vi "Data_PSD_257.vi"() -> ()   [LabVIEW 2020]
uses:
  <vilib>/Utility/error.llb/DialogType.ctl
  <vilib>/Analysis/4window.llb/windowTd.ctl
  <vilib>/Analysis/NI_AALPro.lvlib
  <vilib>/measure/maspectr.llb/Power Spectrum and PSD Export Mode.ctl
  <vilib>/measure/NI_MAPro.lvlib
  <vilib>/sound2/lvsound2.llb/Sound File Info (path).vi
  <vilib>/sound2/lvsound2.llb/Sound File Read (DBL).vi
  <vilib>/sound2/lvsound2.llb/Sound File Read Open.vi
  <vilib>/Analysis/0measdsp.llb/Scaled Time Domain Window (DBL).vi
  <vilib>/measure/maspectr.llb/FFT Power Spectrum and PSD for 1 Chan.vi
panel:
  in  "Stop":bool
  out "Data Cursor":T1
  in  "File Path":path
  out "Max Amplitude":dbl
  out "Frequency Peak":dbl
  out "Signal":waveform(dbl)(graph)
  out "PSD of Signal":cluster{"f0":dbl, "df":dbl, "magnitude":dbl[]}(graph)
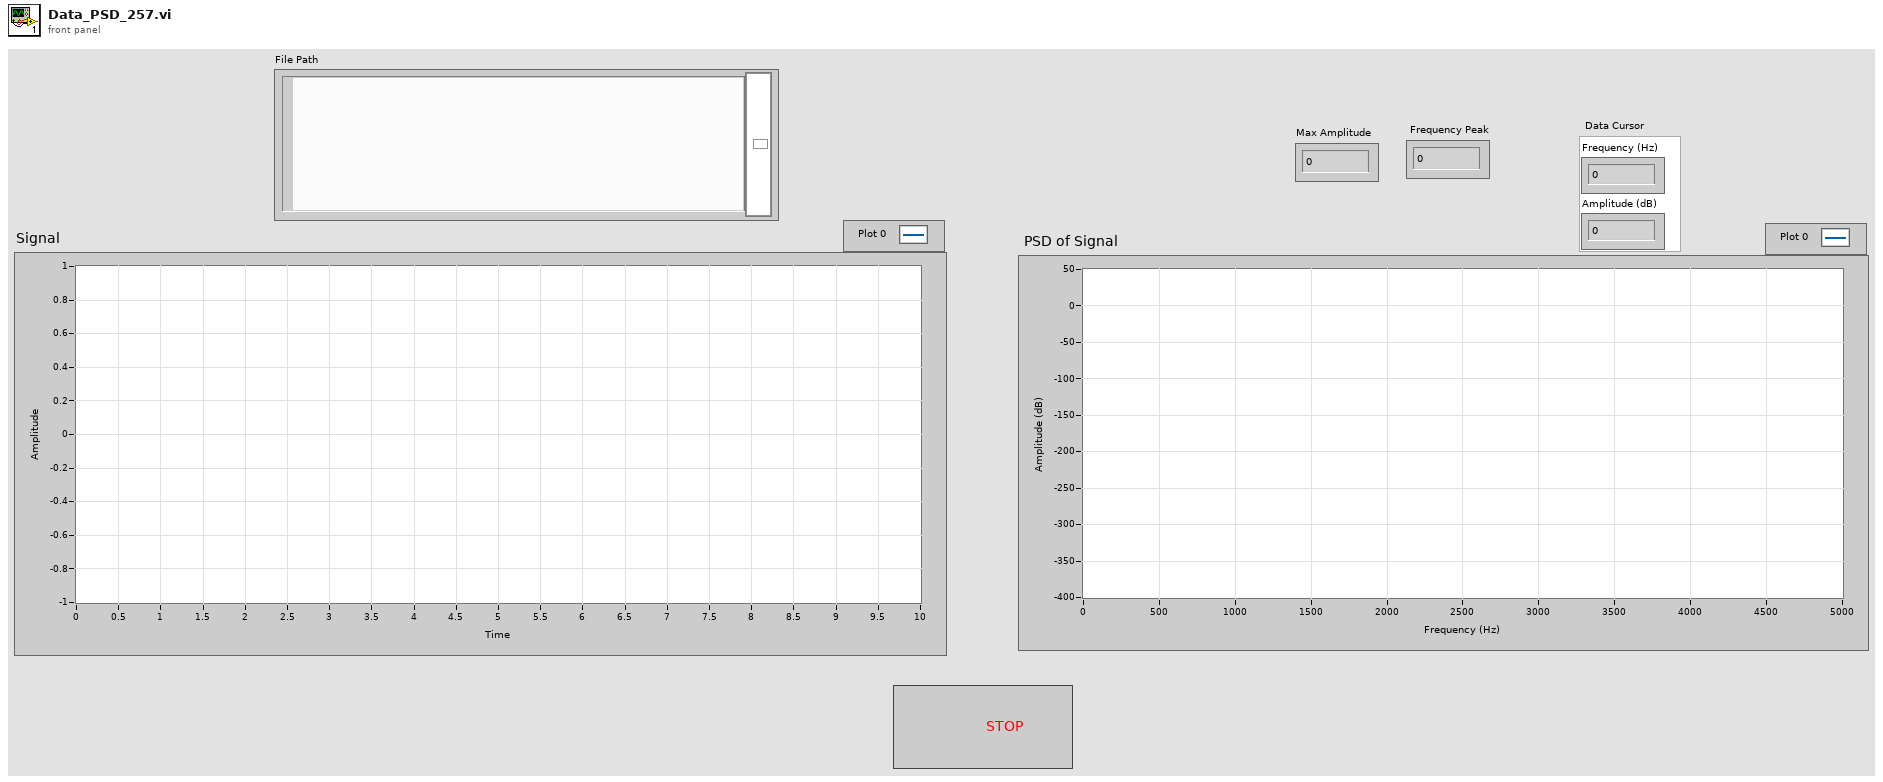
[diagram p1: front panel]
types:
  T1 = cluster{"Frequency (Hz)":dbl, "Amplitude (dB)":dbl}
  T2 = cluster{"Data":dbl[], "ctl":enum16{"Init", "Exit"}}
  T3 = typedef "DialogType.ctl" = u16
  T4 = typedef "NI_AALPro.lvlib/windowTd.ctl" = u32
  T5 = typedef "NI_MAPro.lvlib/Power Spectrum and PSD Export Mode.ctl" = u16
  T6 = typedef "LVPointDoubleTypeDef.ctl" = cluster{"Cursor X":dbl, "Cursor Y":dbl}
  T7 = typedef "Sound File Refnum.ctl" = refnum<file>
  T8 = typedef "LVRangeTypeDef.ctl" = cluster{"Minimum":dbl, "Maximum":dbl, "Increment":dbl, "Minor Increment":dbl, "Start":dbl}
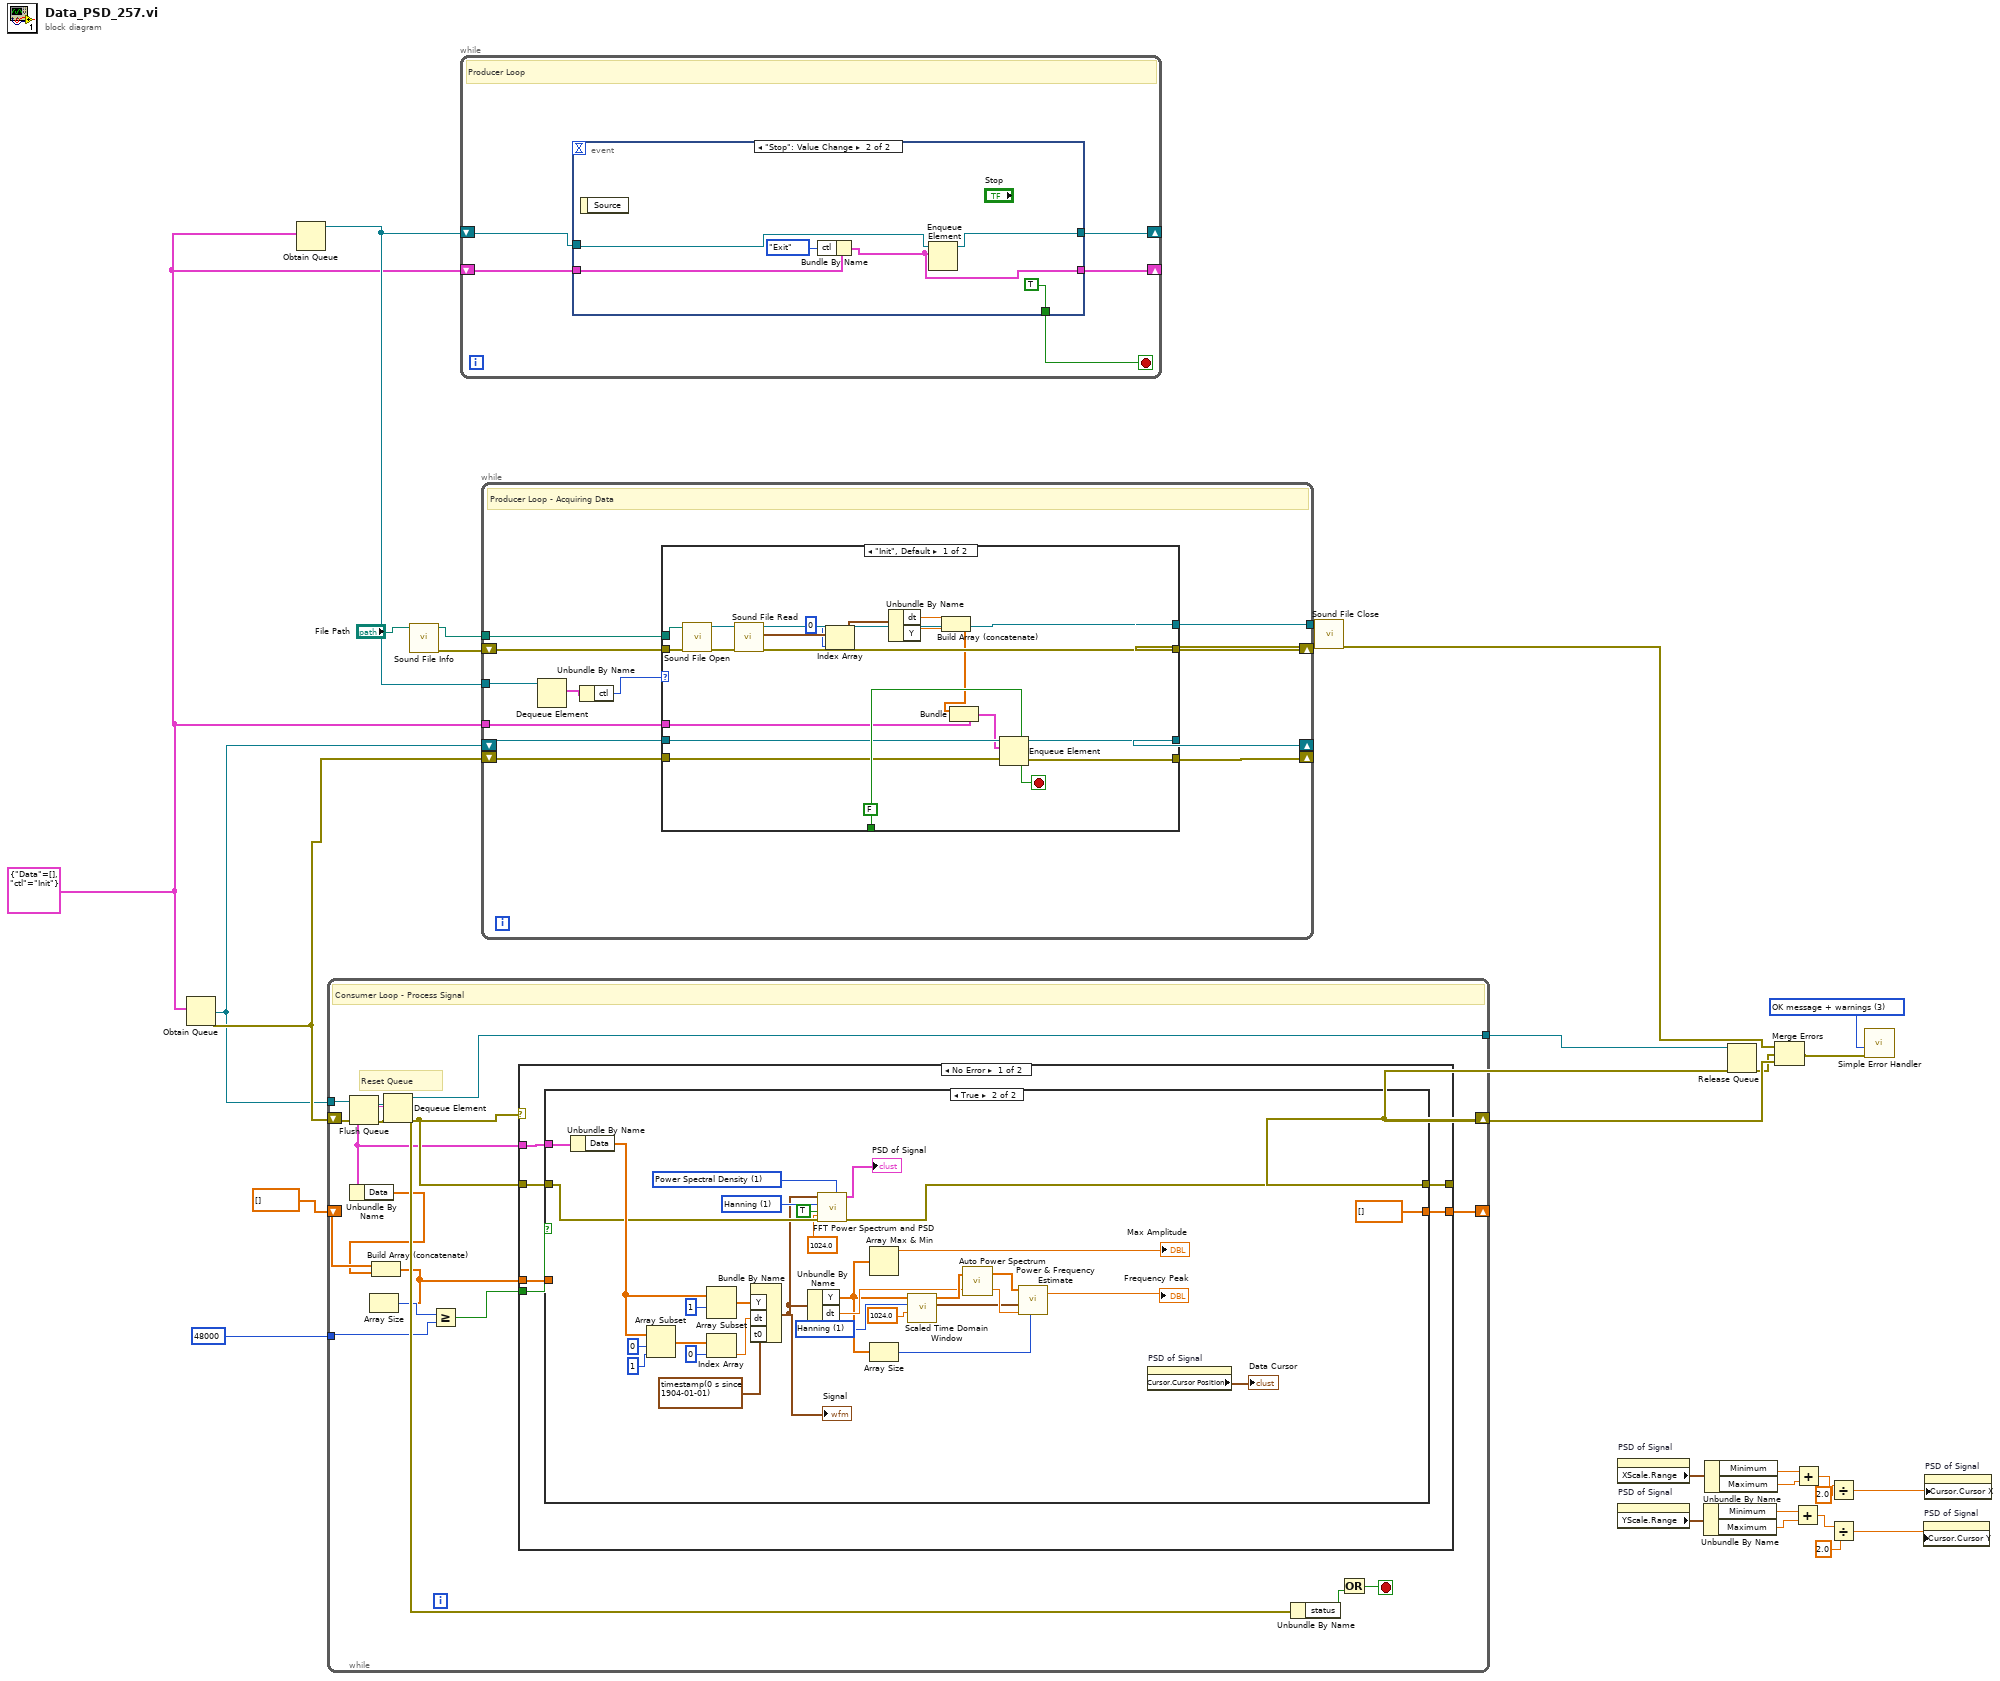
[diagram p0: block diagram]
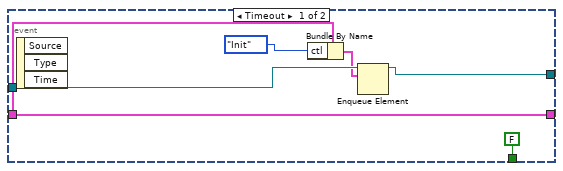
[diagram p2: hidden frame]
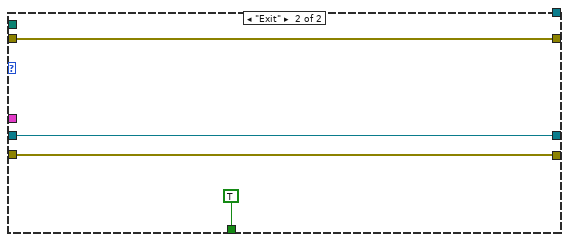
[diagram p3: hidden frame]
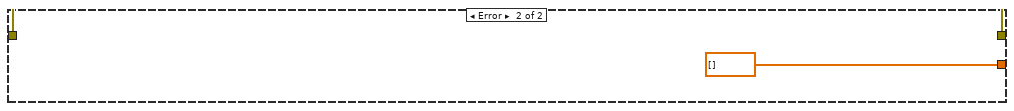
[diagram p5: hidden frame]
diagram:
  w1 = T2 {"Data"=[], "ctl"=enum."Init"}
  w29 = T3 3 items=["no dialog", "OK message", "continue or stop message", "OK message + warnings", "continue/stop + warnings"] ("type of dialog (OK msg:1)")
  n1 = Obtain Queue(element data type=w1) -> (queue out=w18:refnum<queue>, error out=w19:errorcluster)  [unwired: 3 in, 2 out]
  n2 = Obtain Queue(element data type=w1) -> (queue out=w2:refnum<queue>)  [unwired: 4 in, 2 out]
  n3 = while {
    tunnel: w18 -> [w43]
    shift-right: [w46] -> w26
    shift-left: w19 -> [w41]
    tunnel: [w39] -> w27
    tunnel: 48000 -> [w35]
    shift-right: [w31] -> _
    shift-left: dbl[] [] -> [w36]
    stop <- w44 stop-if-true
    # "Reset Queue"
    # "Consumer Loop - Process Signal"
    n4 = Flush Queue(queue=w43, error in (no error)=w41) -> (queue out=w42:refnum<queue>, error out=w40:errorcluster)  [unwired: 1 out]
    n5 = Dequeue Element(queue=w42, error in (no error)=w40) -> (queue out=w39:refnum<queue>, element=w37:T2, error out=w38:errorcluster)  [unwired: 2 out]
    n6 = Unbundle By Name(w37) -> ("Data"=w32:dbl[])
    n7 = Build Array (concatenate)(w36, w32) -> (w30:dbl[])
    n8 = Array Size(array=w30) -> (size(s)=w34:i32)
    n9 = Greater Or Equal?(x=w34, y=w35) -> (x >= y?=w33:bool)
    n10 = case shown="No Error" w38 {
      tunnel: w37 -> [w52 _]
      tunnel: [w47 w87] -> w46
      tunnel: w38 -> [w48 w87]
      tunnel: w33 -> [w51 _]
      tunnel: [w50 dbl[] []] -> w31
      tunnel: w30 -> [w49 _]
      frame No Error {
        n11 = case shown="True" w51 {
          tunnel: w52 -> [_ w67]
          tunnel: [w54 dbl[] []] -> w50
          tunnel: w49 -> [w54 _]
          tunnel: w48 -> [w53 w63]
          tunnel: [w53 w62] -> w47
          frame False {
          }
          frame True {
            w68 = T4 1 items=["Rectangle"=0, "Hanning"=1, "Hamming"=2, "Blackman-Harris"=3, "Exact Blackman"=4, "Blackman"=5, "Flat Top"=6, "4 Term B-Harris "=7, "7 Term B-Harris"=8, "Low Sidelobe"=9, "Blackman Nuttall"=11, "Triangle"=30, "Bartlett-Hanning"=31, "Bohman"=32, "Parzen"=33, "Welch"=34, "Kaiser"=60, "Dolph-Chebyshev"=61, "Gaussian"=62] ("window")
            w69 = T4 1 items=["Rectangle"=0, "Hanning"=1, "Hamming"=2, "Blackman-Harris"=3, "Exact Blackman"=4, "Blackman"=5, "Flat Top"=6, "4 Term B-Harris "=7, "7 Term B-Harris"=8, "Low Sidelobe"=9, "Blackman Nuttall"=11, "Triangle"=30, "Bartlett-Hanning"=31, "Bohman"=32, "Parzen"=33, "Welch"=34, "Kaiser"=60, "Dolph-Chebyshev"=61, "Gaussian"=62] ("window")
            w82 = T5 1 items=["Power Spectrum", "Power Spectral Density"] ("export mode")
            n12 = Unbundle By Name(w67) -> ("Data"=w66:dbl[])
            n13 = Array Subset(array=w66, index=0, length=1) -> (w78:dbl[])
            n14 = Array Subset(array=w66, index=1) -> (w79:dbl[])  [unwired: 1 in]
            n15 = Index Array(array=w78, index=0) -> (element=w76:dbl)
            n16 = Bundle By Name("Y"=w79, "dt"=w76, "t0"=timestamp(0 s since 1904-01-01)) -> (w55:waveform(dbl))  [unwired: 1 in]
            "Signal" <- w55
            n17 = Unbundle By Name(w55) -> ("Y"=w72:dbl[], "dt"=w81:dbl)
            n18 = call-poly <vilib>:"FFT Power Spectrum and PSD.vi"("window parameter"=1024.0, "export mode"=w82, "error in (no error)"=w63, "dB On (F)"=TRUE, "window"=w68, "time signal"=w55) -> ("error out"=w62:errorcluster, "Power Spectrum / PSD"=→"PSD of Signal":cluster{"f0":dbl, "df":dbl, "magnitude":dbl[]})  [unwired: 2 in, 2 out]
            n19 = Array Max & Min(array=w72) -> (max value=→"Max Amplitude":dbl)  [unwired: 3 out]
            n20 = Array Size(array=w72) -> (size(s)=w71:i32)
            n21 = call-poly <vilib>:"Scaled Time Domain Window.vi"("window parameter"=1024.0, "window"=w69, "X"=w72) -> ("window properties"=w70:cluster{"eq noise BW":dbl, "coherent gain":dbl}, "Windowed X"=w84:dbl[])  [unwired: 7 out]
            n22 = call <vilib>:"Auto Power Spectrum.vi"("dt"=w81, "Signal (V)"=w84) -> ("df"=w85:dbl, "Power Spectrum (V^2 rms)"=w73:dbl[])
            n23 = call <vilib>:"Power & Frequency Estimate.vi"("span"=w71, "df"=w85, "window constants"=w70, "Power Spectrum (V^2 rms)"=w73) -> ("est frequency peak"=→"Frequency Peak":dbl)  [unwired: 1 in, 2 out]
            n24 = property on="PSD of Signal" class="WFGraph (strict)"() -> ("Cursor.Cursor Position"=→"Data Cursor":T6)  [unwired: 2 in, 2 out]
          }
        }
      }
      frame Error {
      }
    }
    n25 = Unbundle By Name(w38) -> ("status"=w45:bool)
    n26 = Or(y=w45) -> (x .or. y?=w44:bool)  [unwired: 1 in]
  }
  n27 = call-poly <vilib>:"Sound File Info.vi"("path"="File Path") -> ("error out"=w22:errorcluster, "path out"=w23:path)  [unwired: 7 in, 2 out]
  n28 = while {
    shift-right: [w88] -> _
    shift-left: w1 -> [w91]
    shift-right: [w90] -> _
    shift-left: w2 -> [w92]
    stop <- w89 stop-if-true
    # "Producer Loop"
    n29 = event shown="[1] \"Stop\": Value Change" {
      selector: _ -> [_ _]
      dyn-events: _ -> [_ _]
      timeout: _ -> [_ _]
      tunnel: w92 -> [w98 w102]
      tunnel: w91 -> [w93 w104]
      tunnel: [w95 w101] -> w90
      tunnel: [FALSE TRUE] -> w89
      tunnel: [w93 w99] -> w88
      event Timeout {
        n30 = event-data() -> ()  [unwired: 1 in, 3 out]
        n31 = Bundle By Name(cluster=w93, "ctl"=enum16{"Init", "Exit"}."Init") -> (w96:T2)
        n32 = Enqueue Element(queue=w98, element=w96) -> (queue out=w95:refnum<queue>)  [unwired: 2 in, 2 out]
      }
      event "Stop": Value Change {
        n33 = event-data() -> ()  [unwired: 1 in, 1 out]
        n34 = Bundle By Name(cluster=w104, "ctl"=enum16{"Init", "Exit"}."Exit") -> (w99:T2)
        n35 = Enqueue Element(queue=w102, element=w99) -> (queue out=w101:refnum<queue>)  [unwired: 2 in, 2 out]
      }
    }
  }
  n36 = while {
    shift-right: [w116] -> _
    shift-left: w19 -> [w117]
    shift-right: [w111] -> w20
    shift-left: w22 -> [w113]
    tunnel: w23 -> [w114]
    tunnel: [w112] -> w21
    shift-right: [w109] -> _
    shift-left: w18 -> [w110]
    tunnel: w1 -> [w108]
    tunnel: w2 -> [w105]
    stop <- w115 stop-if-true
    # "Producer Loop - Acquiring Data"
    n37 = Dequeue Element(queue=w105) -> (element=w107:T2)  [unwired: 1 in, 4 out]
    n38 = Unbundle By Name(w107) -> ("ctl"=w106:enum16{"Init", "Exit"})
    n39 = case shown="\"Init\", Default" w106 {
      tunnel: w117 -> [w136 w138]
      tunnel: [w135 w138] -> w116
      tunnel: [FALSE TRUE] -> w115
      tunnel: w114 -> [w134 _]
      tunnel: w113 -> [w132 w137]
      tunnel: [w130 _] -> w112
      tunnel: [w126 w137] -> w111
      tunnel: w110 -> [w122 w139]
      tunnel: [w120 w139] -> w109
      tunnel: w108 -> [w119 _]
      frame "Init", Default {
        n40 = call-poly <vilib>:"Sound File Open.vi"("error in (no error)"=w132, "path"=w134) -> ("error out"=w131:errorcluster, "sound file refnum"=w133:T7)  [unwired: 8 in]
        n41 = call-poly <vilib>:"Sound File Read.vi"("error in (no error)"=w131, "sound file refnum"=w133) -> ("error out"=w126:errorcluster, "data"=w129:waveform(dbl)[], "sound file refnum out"=w130:T7)  [unwired: 5 in, 2 out]
        n42 = Index Array(array=w129, index=0) -> (element=w127:waveform(dbl))
        n43 = Unbundle By Name(w127) -> ("dt"=w125:dbl, "Y"=w124:dbl[])
        n44 = Build Array (concatenate)(w125, w124) -> (w123:dbl[])
        n45 = Bundle(cluster=w119, "Data"=w123) -> (w121:T2)  [unwired: 1 in]
        n46 = Enqueue Element(queue=w122, element=w121, error in (no error)=w136) -> (queue out=w120:refnum<queue>, error out=w135:errorcluster)  [unwired: 2 out]
      }
      frame "Exit" {
      }
    }
  }
  n47 = call <vilib>:"Sound File Close.vi"("error in (no error)"=w20, "sound file refnum"=w21) -> ("error out"=w17:errorcluster)  [unwired: 9 in]
  n48 = property on="PSD of Signal" class="WFGraph (strict)"() -> ("XScale.Range"=w14:T8)  [unwired: 2 in, 2 out]
  n49 = property on="PSD of Signal" class="WFGraph (strict)"() -> ("YScale.Range"=w13:T8)  [unwired: 2 in, 2 out]
  n50 = Unbundle By Name(w13) -> ("Minimum"=w6:dbl, "Maximum"=w5:dbl)
  n51 = Unbundle By Name(w14) -> ("Minimum"=w12:dbl, "Maximum"=w11:dbl)
  n52 = Release Queue(queue=w27, error in (no error)=w26) -> (error out=w25:errorcluster)  [unwired: 1 in, 2 out]
  n53 = Merge Errors(w17, w25, w26) -> (w28:errorcluster)
  n54 = Add(x=w6, y=w5) -> (x+y=w8:dbl)
  n55 = Add(x=w12, y=w11) -> (x+y=w9:dbl)
  n56 = Divide(x=2.0 ("y"), y=w9) -> (x/y=w3:dbl)
  n57 = Divide(x=w8, y=2.0) -> (x/y=w4:dbl)
  n58 = call <vilib>:"Simple Error Handler.vi"("type of dialog (OK msg:1)"=w29, "error in (no error)"=w28) -> ()  [unwired: 8 out]
  n59 = property on="PSD of Signal" class="WFGraph (strict)"("Cursor.Cursor Y"=w4) -> ()  [unwired: 2 in, 2 out]
  n60 = property on="PSD of Signal" class="WFGraph (strict)"("Cursor.Cursor X"=w3) -> ()  [unwired: 2 in, 2 out]
